vi "file pgm.vi"(8 "max_val":i32, 9 "gamma":dbl=2.0, 10 "Path":path=path "C:/Users/Green Beret/Documents/Visual Studio 2012/Projects/LightPipes/LightPipes/lp12src/LabView/images/path.pgm", 11 "field":T1) -> (2 "path pgm":string, 3 "field out":T1)   [LabVIEW 2012]
doc: "__declspec(dllexport) void file_pgm(double gamma, int max_val, FIELD* field);\n\n__declspec(dllexport) void file_pgm(FIELD* field, const char* path, double gamma, int max_val);"
uses:
  Lightpipes.dll
  LightPipes.lvlib
panel:
  out "error out":errorcluster
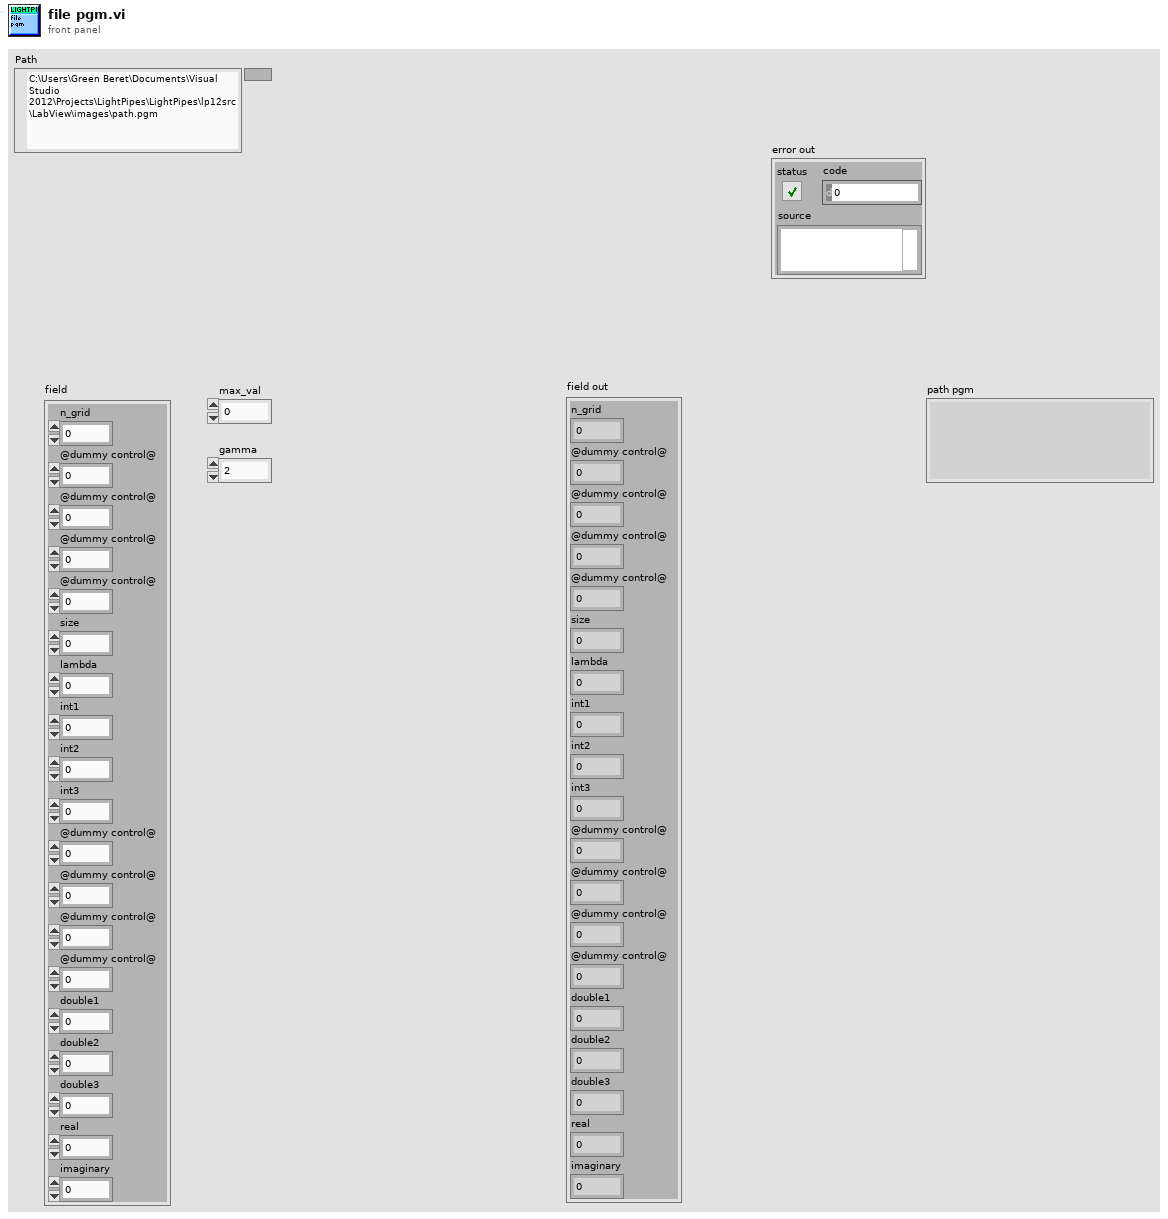
[diagram p1: front panel]
types:
  T1 = cluster{"n_grid":i32, "@dummy control@":i8, "@dummy control@":i8, "@dummy control@":i8, "@dummy control@":i8, "size":dbl, "lambda":dbl, "int1":i32, "int2":i32, "int3":i32, "@dummy control@":i8, "@dummy control@":i8, "@dummy control@":i8, "@dummy control@":i8, "double1":dbl, "double2":dbl, "double3":dbl, "real":u32, "imaginary":u32}
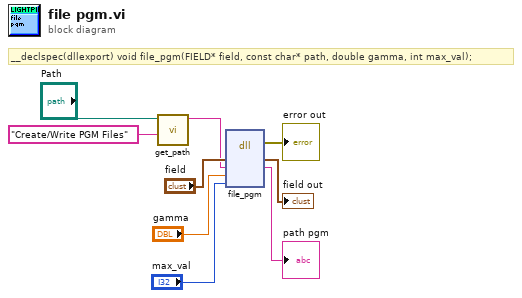
[diagram p0: block diagram]
diagram:
  # "__declspec(dllexport) void file_pgm(FIELD* field, const char* path, double gamma, int max_val);"
  n1 = call "get_path.vi"("Message Prompt"="Create/Write PGM Files", "Path In"="Path") -> ("Path out"=w5:string)  [unwired: 9 in]
  n2 = dll-call lib="C:/Users/Tri/Documents/Gerchberg/LightPipes.*" fn="file_pgm"("field"="field", "path"=w5, "gamma"="gamma", "max_val"="max_val") -> (error out=→"error out":errorcluster, "field"=→"field out":T1, "path"=→"path pgm":string)  [unwired: 6 in, 1 out]
